vi "ProyectoFinalIV.vi"() -> ()   [LabVIEW 2020]
uses:
  <vilib>/Instr/_visa.llb/VISA Configure Serial Port (Instr).vi
panel:
  out "concatenated string 2":string
  out "read buffer":string
  in  "stop":bool
  in  "Settings":T1={"Objects"=0, "Threshold"=128, "Reject Border"=FALSE, "Fill Holes"=FALSE, "Min Object Size"=FALSE, "Min Size"=3, "Max Object Size"=FALSE, "Max Size"=100, "Show Search Area"=FALSE, "Show Center"=TRUE, "Show Bounding Box"=TRUE} {"Objects" items=["Bright Objects", "Dark Objects"]; "Threshold" min=1 max=999999999 step=1; "Max Size" min=1 max=999999999 step=1; "Min Size" min=1 max=999999999 step=1}
  out "Objects":T2(array[cluster]) {"Aspect Ratio" format="%.2f"; "Orientation" format="%.2f"; "Area" format="%.2f"; "Object Center"."Y" format="%.2f"; "Object Center"."X" format="%.2f"}
  in  "Tab Control":T3(tab)
  out "Humedad":dbl(knob) scale=0.0..100.0
  in  "bomba btn":bool
  in  "ventilador btn":bool
  in  "valvula btn":bool
  out "bomba":bool
  out "ventilador":bool
  in  "Disabled":T4(ring)
  out "válvula":bool
  out "Waveform Graph":dbl[](graph)
  out "Temperatura invernadero":dbl(slide) scale=0.0..100.0
  out "ml en tanque":dbl(slide) scale=0.0..1000.0
  in  "VISA resource name":refnum<visa-resource-name>
  out "number":dbl
  in  "Alto de la planta.":string
  in  "Guardar la siguiente  imagen?.":bool
  out "fecha de captura":string
  in  "Etapa de desarrollo":string
  in  "Capturar imagen.":bool
  out "Capturada":T5(plugin-control)
  out "Number of Objects":i32
  out "concatenated string":string
  in  "Direccion":path=path "C:/Users/Rodol/Pictures/IV_Invernadero/vie., 16 de jun. de 2023.jpg" caption="Image Path"
  out "Image Out":T5(plugin-control)
  # "Equipo 8: invernadero con  vision artificial."
  # "actuadores"
  # "Ver foto"
  # "Accionamiento manual"
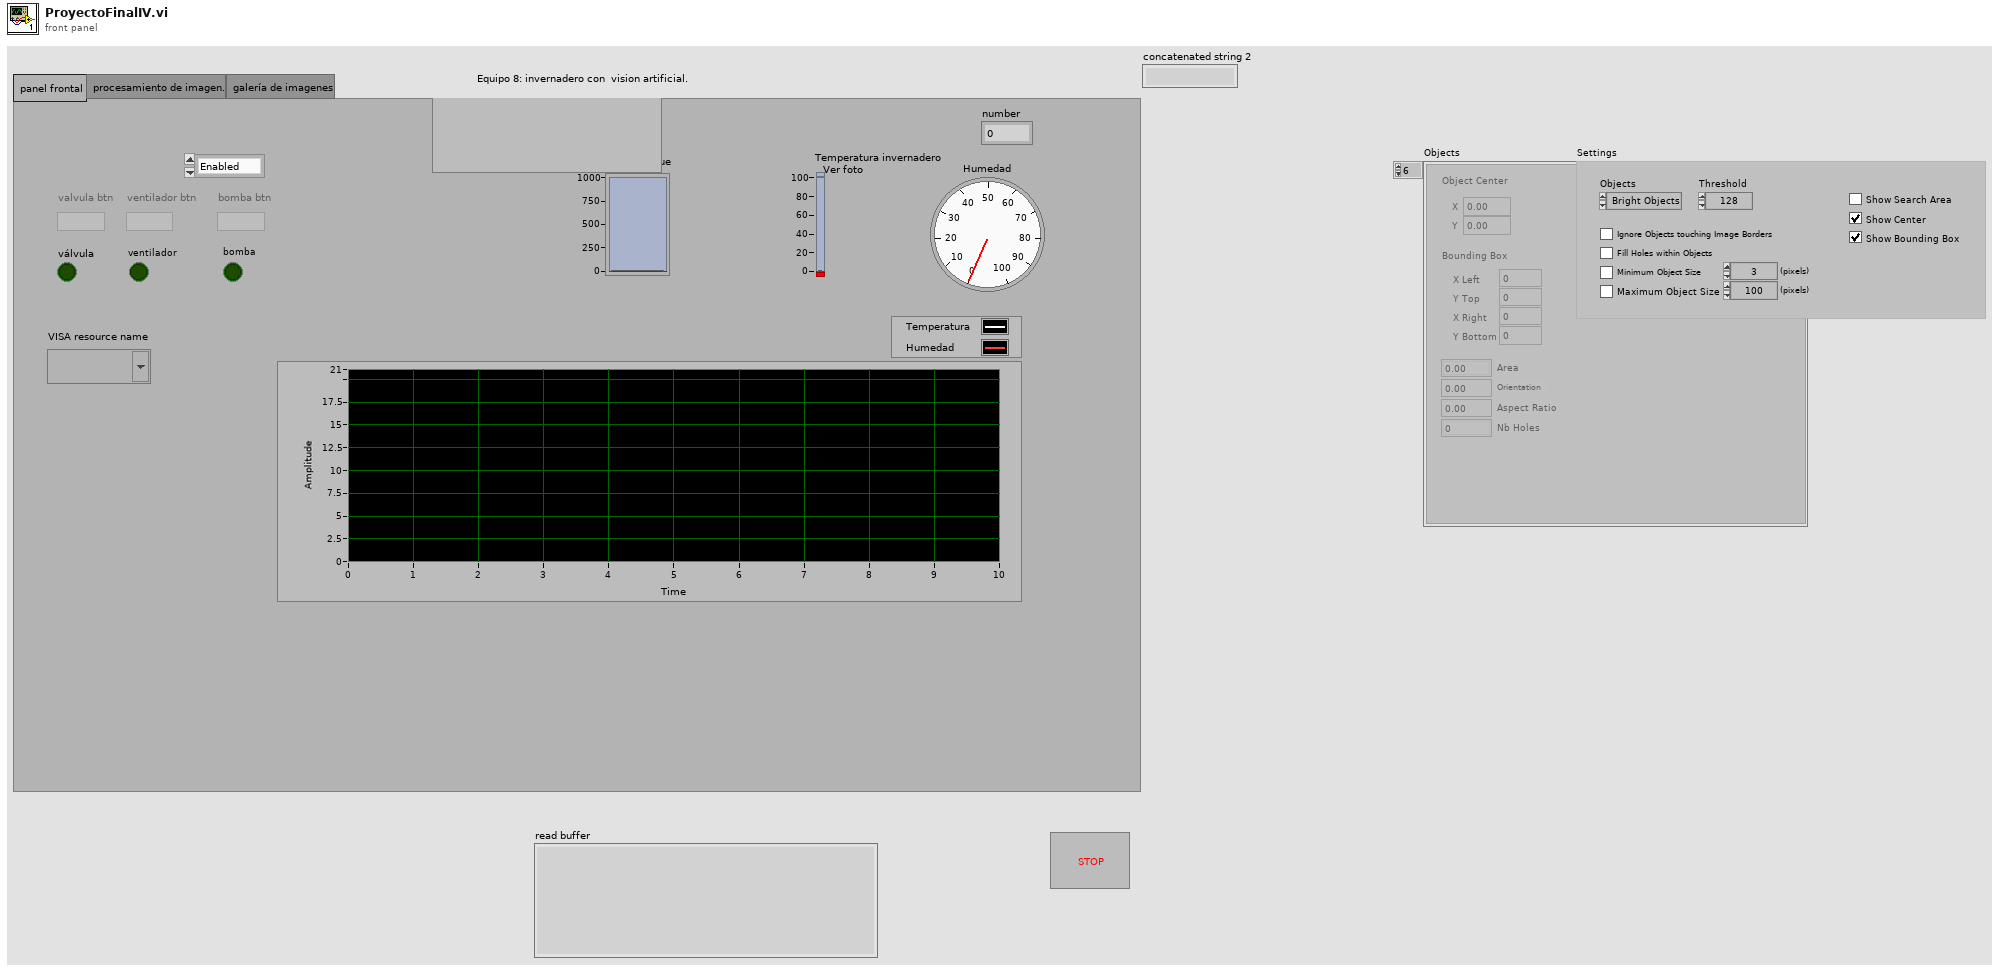
[diagram p1: front panel]
types:
  T1 = cluster{"Objects":u16, "Threshold":i32, "Reject Border":bool, "Fill Holes":bool, "Min Object Size":bool, "Min Size":i32, "Max Object Size":bool, "Max Size":i32, "Show Search Area":bool, "Show Center":bool, "Show Bounding Box":bool}
  T2 = cluster{"Object Center":cluster{"X":sgl, "Y":sgl}, "Bounding Box":cluster{"X Left":i32, "Y Top":i32, "X Right":i32, "Y Bottom":i32}, "Area":sgl, "Orientation":sgl, "Aspect Ratio":sgl, "Nb Holes":i32}[]
  T3 = enum32{"panel frontal", "procesamiento de imagen.", "galería de imagenes"}
  T4 = enum8{"Enabled", "Disabled", "Disabled and Grayed Out"}
  T5 = typedef "IMAQ Image.ctl" = refnum<image>
  T6 = enum16{"open", "replace", "create", "open or create", "replace or create", "replace or create with confirmation"}
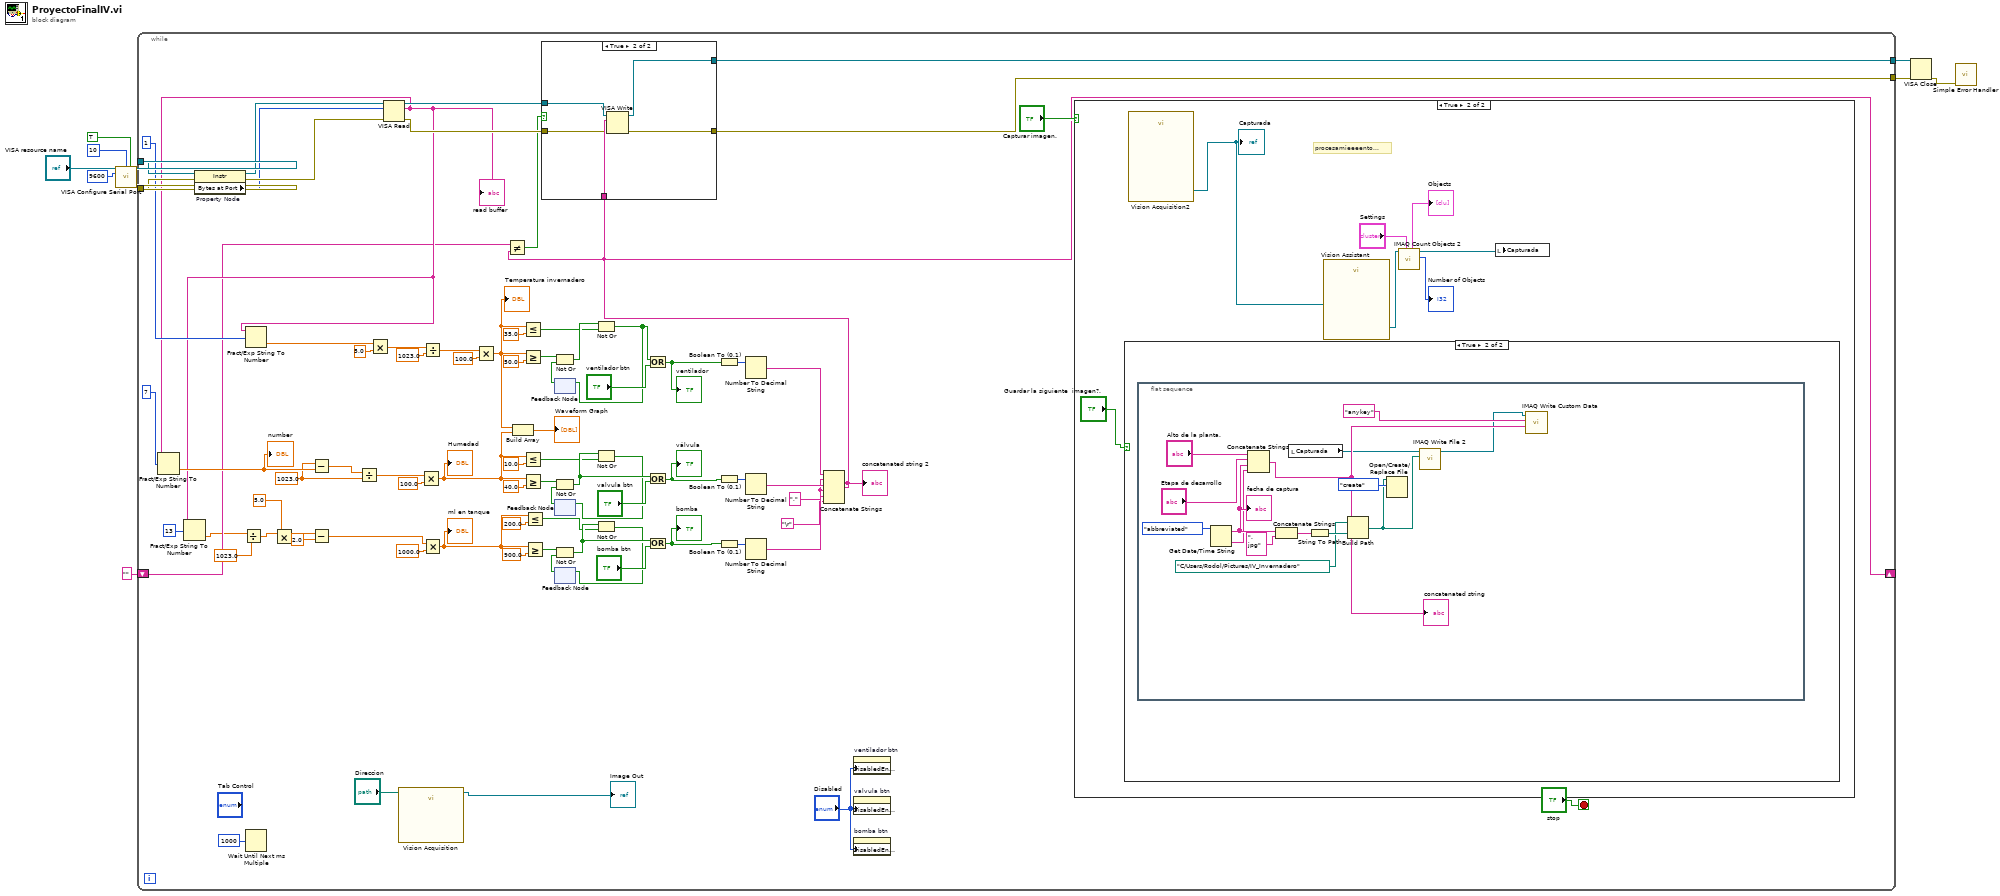
[diagram p0: block diagram]
diagram:
  n1 = call-poly "VISA Configure Serial Port"("VISA resource name"="VISA resource name", "termination char\n(0xA = '\\n' = LF)"=u8 10 ("termination char\n(0xA = '\\n' = LF)"), "Enable Termination\nChar (T)"=TRUE ("Enable Termination\nChar (T)"), "baud rate (9600)"=u32 9600) -> ("VISA resource name out"=w5:refnum<visa-resource-name>, "error out"=w6:errorcluster)  [unwired: 10 in]
  n2 = while {
    tunnel: w6 -> [w88]
    tunnel: w5 -> [w90]
    tunnel: [w30] -> w3
    tunnel: [w29] -> w2
    shift-right: [w21] -> _
    shift-left: "" -> [w22]
    stop <- "stop" stop-if-true
    w48 = "," ("string")
    w39 = 1023.0 ("x")
    n3 = property on="Property Node" class="Instr"(reference=w90, error in=w88) -> (reference out=w89:refnum<visa-resource-name>, error out=w87:errorcluster, "Bytes at Port"=w81:u32)
    n4 = Wait Until Next ms Multiple(millisecond multiple=u32 1000) -> ()  [unwired: 1 out]
    n5 = VISA Read(VISA resource name=w89, byte count=w81, error in (no error)=w87) -> (VISA resource name out=w32:refnum<visa-resource-name>, read buffer=w28:string, error out=w31:errorcluster)  [unwired: 1 out]
    "read buffer" <- w28
    n6 = Fract/Exp String To Number(string=w28, offset=7) -> (number=w52:dbl)  [unwired: 2 in, 1 out]
    "number" <- w52
    n7 = Fract/Exp String To Number(string=w28, offset=13) -> (number=w17:dbl)  [unwired: 2 in, 1 out]
    n8 = Divide(x=w17, y=1023.0) -> (x/y=w15:dbl)
    n9 = Fract/Exp String To Number(string=w28, offset=1) -> (number=w49:dbl)  [unwired: 2 in, 1 out]
    n10 = Multiply(x=w15, y=5.0) -> (x*y=w13:dbl)
    n11 = Subtract(x=w39, y=w52) -> (x-y=w53:dbl)
    n12 = Subtract(x=w13, y=2.0) -> (x-y=w11:dbl)
    n13 = Divide(x=w53, y=w39) -> (x/y=w54:dbl)
    n14 = Multiply(x=w49, y=5.0) -> (x*y=w50:dbl)
    n15 = call "Vision Acquisition"("Image Path"="Direccion") -> ("Image Out"=→"Image Out":T5)  [unwired: 25 in, 1 out]
    n16 = Multiply(x=w54, y=100.0) -> (x*y=w70:dbl)
    "Humedad" <- w70
    n17 = Divide(x=w50, y=1023.0) -> (x/y=w51:dbl)
    n18 = Multiply(x=w11, y=1000.0) -> (x*y=w66:dbl)
    "ml en tanque" <- w66
    n19 = Multiply(x=w51, y=100.0) -> (x*y=w69:dbl)
    "Temperatura invernadero" <- w69
    n20 = Build Array(w69, w70) -> (→"Waveform Graph":dbl[])
    n21 = Less Or Equal?(x=w69, y=35.0) -> (x <= y?=w58:bool)
    n22 = Greater Or Equal?(x=w69, y=50.0) -> (x >= y?=w57:bool)
    n23 = Less Or Equal?(x=w70, y=10.0) -> (x <= y?=w61:bool)
    n24 = Greater Or Equal?(x=w70, y=40.0) -> (x >= y?=w60:bool)
    n25 = Less Or Equal?(x=w66, y=200.0) -> (x <= y?=w64:bool)
    n26 = Greater Or Equal?(x=w66, y=900.0) -> (x >= y?=w63:bool)
    n27 = feedback #1() -> (w56:bool)  [unwired: 1 in]
    n28 = Not Or(1:w56, 2:w57) -> (0:w80:bool)
    n29 = feedback #2() -> (w59:bool)  [unwired: 1 in]
    n30 = Not Or(1:w59, 2:w60) -> (0:w79:bool)
    n31 = feedback #3() -> (w62:bool)  [unwired: 1 in]
    n32 = Not Or(1:w62, 2:w63) -> (0:w78:bool)
    n33 = Not Or(1:w58, 2:w80) -> (0:w24:bool)
    n34 = feedback-in #1(w24) -> ()
    n35 = Not Or(1:w61, 2:w79) -> (0:w25:bool)
    n36 = feedback-in #2(w25) -> ()
    n37 = Not Or(1:w64, 2:w78) -> (0:w26:bool)
    n38 = feedback-in #3(w26) -> ()
    n39 = Or(x=w24, y="ventilador btn") -> (x .or. y?=w20:bool)
    "ventilador" <- w20
    n40 = Or(x=w79, y="valvula btn") -> (x .or. y?=w19:bool)
    "válvula" <- w19
    n41 = Or(x=w78, y="bomba btn") -> (x .or. y?=w18:bool)
    "bomba" <- w18
    n42 = Boolean To (0,1)(Boolean=w20) -> (0, 1=w72:i16)
    n43 = Boolean To (0,1)(Boolean=w19) -> (0, 1=w73:i16)
    n44 = Boolean To (0,1)(Boolean=w18) -> (0, 1=w74:i16)
    n45 = Number To Decimal String(number=w72) -> (decimal integer string=w75:string)  [unwired: 1 in]
    n46 = Number To Decimal String(number=w73) -> (decimal integer string=w76:string)  [unwired: 1 in]
    n47 = Number To Decimal String(number=w74) -> (decimal integer string=w77:string)  [unwired: 1 in]
    n48 = Concatenate Strings(w75, w48, w76, w48, w77, "\r") -> (w21:string)
    "concatenated string 2" <- w21
    n49 = Not Equal?(x=w22, y=w21) -> (x != y?=w23:bool)
    n50 = case shown="True" w23 {
      tunnel: w21 -> [_ w97]
      tunnel: w32 -> [w92 w96]
      tunnel: w31 -> [w91 w95]
      tunnel: [w92 w94] -> w30
      tunnel: [w91 w93] -> w29
      frame False {
      }
      frame True {
        n51 = VISA Write(VISA resource name=w96, write buffer=w97, error in (no error)=w95) -> (VISA resource name out=w94:refnum<visa-resource-name>, error out=w93:errorcluster)  [unwired: 1 out]
      }
    }
    n52 = property on="ventilador btn" class="Bool (strict)"("DisabledEnum"="Disabled") -> ()  [unwired: 2 in, 2 out]
    n53 = property on="valvula btn" class="Bool (strict)"("DisabledEnum"="Disabled") -> ()  [unwired: 2 in, 2 out]
    n54 = property on="bomba btn" class="Bool (strict)"("DisabledEnum"="Disabled") -> ()  [unwired: 2 in, 2 out]
    n55 = case shown="True" "Capturar imagen." {
      frame False {
      }
      frame True {
        # "procesamieeeento..."
        n56 = case shown="True" "Guardar la siguiente  imagen?." {
          frame False {
          }
          frame True {
            n57 = flat-sequence {
              frame #0 {
                n58 = Get Date/Time String(date format (0)=enum16{"short", "long", "abbreviated"}."abbreviated") -> (date string=w110:string, time string=w109:string)  [unwired: 2 in]
                "fecha de captura" <- w110
                n59 = Concatenate Strings("Alto de la planta.", "Etapa de desarrollo", w110, w109) -> (w108:string)
                "concatenated string" <- w108
                n60 = Concatenate Strings(w110, ".jpg" ("string")) -> (w119:string)
                n61 = local read "Capturada"() -> (w107:T5)
                n62 = String To Path(string=w119) -> (path=w118:path)
                n63 = Build Path(base path=path "C:/Users/Rodol/Pictures/IV_Invernadero", name or relative path=w118) -> (appended path=w115:path)
                n64 = Open/Create/Replace File(file path (use dialog)=w115, operation (0:open)=T6."create") -> ()  [unwired: 4 in, 3 out]
                n65 = call-poly "IMAQ Write File 2"("File Path"=w115, "Image"=w107) -> ("Image Out (duplicate)"=w105:T5)  [unwired: 8 in, 1 out]
                n66 = call "IMAQ Write Custom Data"("Custom Data In"=w108, "Key"="anykey", "Image"=w105) -> ()  [unwired: 7 in, 2 out]
              }
            }
          }
        }
        n67 = call "Vision Acquisition2"() -> ("Image Out"=w100:T5)  [unwired: 26 in, 1 out]
        "Capturada" <- w100
        n68 = call "Vision Assistant"("Image In"=w100) -> ("Image Out"=w104:T5)  [unwired: 25 in, 1 out]
        n69 = call "IMAQ Count Objects 2"("Settings"="Settings", "Image"=w104) -> ("Number of Objects"=→"Number of Objects":i32, "Image Out"=w99:T5, "Objects"=→"Objects":T2)  [unwired: 5 in, 2 out]
        n70 = local write "Capturada"(w99) -> ()
      }
    }
  }
  n71 = VISA Close(VISA resource name=w3, error in (no error)=w2) -> (error out=w4:errorcluster)
  n72 = call <vilib>:"Simple Error Handler.vi"("error in (no error)"=w4) -> ()  [unwired: 4 in, 5 out]
